vi "WS1050 Delta C_RTZ Ver1.0.vi"(8 "error in (no error)":errorcluster, 9 "CMin_C1":dbl, 11 "Bank C1":string[](array[string])) -> (0 "error out":errorcluster, 2 "C1_RTZ":string[](array[string]), 3 "Delta C(pF)":string[](array[string]))   [LabVIEW 2017]
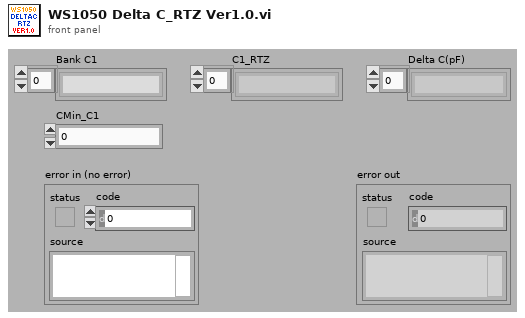
[diagram p1: front panel]
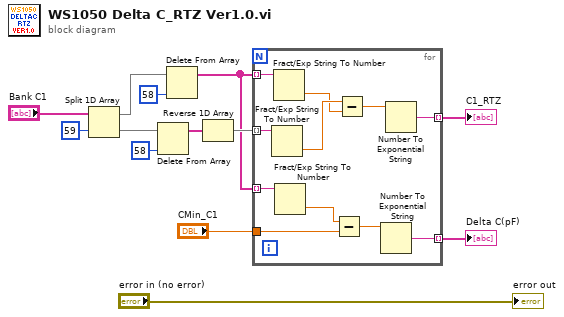
[diagram p0: block diagram]
diagram:
  n1 = Split 1D Array(array="Bank C1", index=59) -> (first subarray=w12:string[], second subarray=w10:string[])
  n2 = Delete From Array(array=w10, index=58) -> (array with subset deleted=w8:string[])  [unwired: 1 in, 1 out]
  n3 = Delete From Array(array=w12, index=58) -> (array with subset deleted=w4:string[])  [unwired: 1 in, 1 out]
  n4 = Reverse 1D Array(array=w8) -> (reversed array=w7:string[])
  n5 = for {
    tunnel: w4 -> [w24] mode=indexing
    tunnel: w7 -> [w23] mode=indexing
    tunnel: [w19] -> w5 mode=indexing
    tunnel: w4 -> [w18] mode=indexing
    tunnel: "CMin_C1" -> [w16]
    tunnel: [w14] -> w2 mode=indexing
    n6 = Fract/Exp String To Number(string=w23) -> (number=w22:dbl)  [unwired: 3 in, 1 out]
    n7 = Fract/Exp String To Number(string=w24) -> (number=w21:dbl)  [unwired: 3 in, 1 out]
    n8 = Fract/Exp String To Number(string=w18) -> (number=w17:dbl)  [unwired: 3 in, 1 out]
    n9 = Subtract(x=w17, y=w16) -> (x-y=w15:dbl)
    n10 = Subtract(x=w22, y=w21) -> (x-y=w20:dbl)
    n11 = Number To Exponential String(number=w15) -> (E-format string=w14:string)  [unwired: 3 in]
    n12 = Number To Exponential String(number=w20) -> (E-format string=w19:string)  [unwired: 3 in]
  }
  "C1_RTZ" <- w5
  "Delta C(pF)" <- w2
  "error out" <- "error in (no error)"
